vi "Create Test Configuration.vi"() -> (0 "error out":errorcluster, 1 "Names":string[](array[string]), 2 "Line Array":T1[](array[typedef]), 3 "Module Configuration":refnum<class "Multiplexer configuration.lvclass">, 4 "Channels":refnum<class "TBM channel.lvclass">[](array[class]), 5 "instance identifier":string)   [LabVIEW 2021, in "Multiplexer tests.lvlib"]
doc: "This VI creates a standard test configuration for other unit tests. It currently creates and adds one line with every datatype to the module configuration."
uses:
  Multiplexer tests.lvlib
  configuration/Multiplexer configuration.lvclass
  C:/Program Files (x86)/National Instruments/LabVIEW 2021/vi.lib/NI/Configuration Framework/serializable configuration/NISE_CEF_serializable configuration.lvclass
  configuration/Line.ctl
  <vilib>/NI/Tag Bus Module Framework/channel/TBM channel.lvclass
  <vilib>/NI/Tag Bus Module Framework/channel/channel classification.ctl
  <vilib>/NI/Tag Bus/tag/Data Type.ctl
  configuration/Multiplexer configuration.lvclass/Multiplexer configuration.ctl
  configuration/Write Scale.vi
  <vilib>/NI/Configuration Framework/serializable configuration/NISE_CEF_serializable configuration.lvclass
  <vilib>/NI/Tag Bus/tag/tag descriptor.lvclass
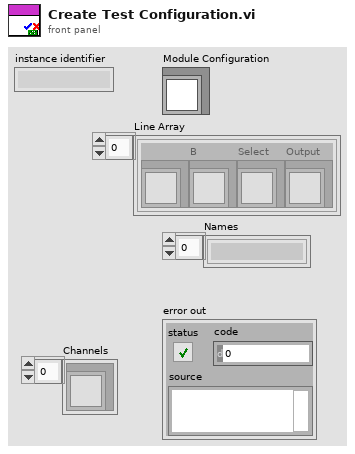
[diagram p1: front panel]
types:
  T1 = typedef "Multiplexer configuration.lvclass/Line.ctl" = cluster{"A":refnum<class "TBM channel.lvclass">, "B":refnum<class "TBM channel.lvclass">, "Select":refnum<class "TBM channel.lvclass">, "Output":refnum<class "TBM channel.lvclass">}
  T2 = typedef "tag bus.lvlib/tag descriptor.lvclass/Data Type.ctl" = enum16{"Double", "Single", "I64", "I32", "I16", "I8", "U64", "U32", "U16", "U8", "Boolean", "String", "Array of Double", "Array of Single", "Array of I64", "Array of I32", "Array of I16", "Array of I8", "Array of U64", "Array of U32", "Array of U16", "Array of U8", "Array of Boolean", "Array of String"}
  T3 = typedef "TBM channel.lvclass/channel classification.ctl" = enum16{"input data", "output data", "processing parameter", "processing result"}
  T4 = cluster{"[0]":refnum<class "TBM channel.lvclass">, "[1]":refnum<class "TBM channel.lvclass">, "[2]":refnum<class "TBM channel.lvclass">, "[3]":refnum<class "TBM channel.lvclass">}
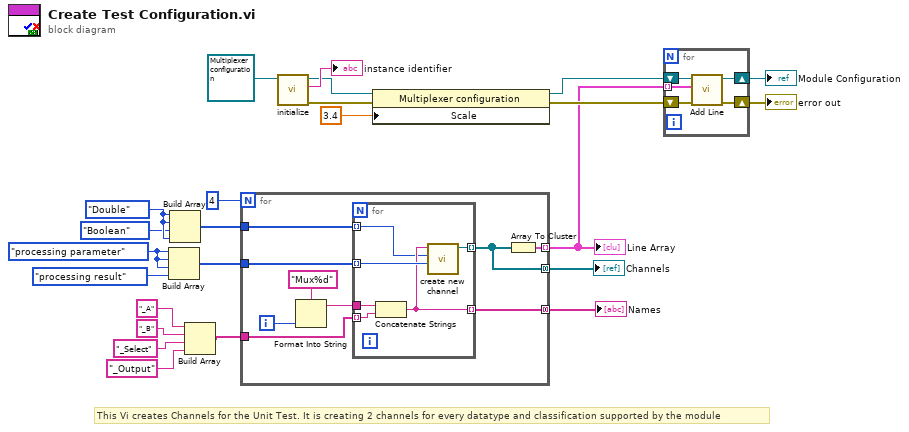
[diagram p0: block diagram]
diagram:
  w3 = Data_Type."Double" ("data type")
  w9 = channel_classification."processing parameter" ("channel classification")
  # "This Vi creates Channels for the Unit Test. It is creating 2 channels for every datatype and classification supported by the module"
  n1 = Build Array(w9, w9, w9, channel_classification."processing result" ("element")) -> (w8:T3[])
  n2 = Build Array(w3, w3, Data_Type."Boolean" ("element"), w3) -> (w1:T2[])
  n3 = Build Array("_A" ("format string"), "_B" ("element"), "_Select" ("element"), "_Output" ("element")) -> (w7:string[])
  n4 = for {
    N: 4 -> [_]
    tunnel: [w32] -> w18 mode=indexing
    tunnel: [w31] -> w20 mode=concatenating
    tunnel: [w33] -> w14 mode=concatenating
    tunnel: w8 -> [w30]
    tunnel: w7 -> [w26]
    tunnel: w1 -> [w25]
    i -> [w29]
    n5 = Format Into String(format string="Mux%d", w29) -> (resulting string=w28:string)  [unwired: 2 in, 1 out]
    n6 = for {
      tunnel: w30 -> [w39] mode=indexing
      tunnel: [w38] -> w33 mode=indexing
      tunnel: [w35] -> w31 mode=indexing
      tunnel: w26 -> [w37] mode=indexing
      tunnel: w28 -> [w36]
      tunnel: w25 -> [w34] mode=indexing
      n7 = Concatenate Strings(w36, w37) -> (w35:string)
      n8 = call <vilib>:"create new channel.vi"("channel classification"=w39, "data type"=w34, "channel name"=w35) -> ("channel"=w38:refnum<class "TBM channel.lvclass">)  [unwired: 8 in]
    }
    n9 = Array To Cluster(array=w33) -> (cluster=w32:T4)
  }
  "Names" <- w20
  "Line Array" <- w18
  "Channels" <- w14
  n10 = call <vilib>:"initialize.vi"("configuration in"=refnum<class "Multiplexer configuration.lvclass"> refnum ("tag bus configurable plugin module configuration")) -> ("error out"=w22:errorcluster, "identifier"=→"instance identifier":string, "configuration out"=w19:refnum<class "Multiplexer configuration.lvclass">)  [unwired: 8 in]
  n11 = property class="Multiplexer configuration"(reference=w19, error in=w22, "Scale"=3.4) -> (reference out=w15:refnum<class "Multiplexer configuration.lvclass">, error out=w21:errorcluster)
  n12 = for {
    tunnel: w18 -> [w40] mode=indexing
    shift-right: [w43] -> w17
    shift-left: w15 -> [w44]
    shift-right: [w41] -> w24
    shift-left: w21 -> [w42]
    n13 = call "Add Line.vi"("error in"=w42, "Line"=w40, "Multiplexer configuration in"=w44) -> ("error out"=w41:errorcluster, "Multiplexer configuration out"=w43:refnum<class "Multiplexer configuration.lvclass">)  [unwired: 6 in, 1 out]
  }
  "error out" <- w24
  "Module Configuration" <- w17
